vi "Send.vi"(9 "Nested Error":errorcluster, 10 "Nested Actor":refnum<class "Actor.lvclass">) -> (3 "Actor Last Ack Msg Strategy out":refnum<class "Actor Last Ack Msg Strategy.lvclass">)   [LabVIEW 2021, in "Actor Last Ack.lvlib" / "Actor Last Ack Msg Strategy.lvclass"]
uses:
  Actor Last Ack Msg Strategy.lvclass
  LVCAM/Actor/Actor.lvclass
  Actor Last Ack Msg Strategy.lvclass/Actor Last Ack Msg Strategy.ctl
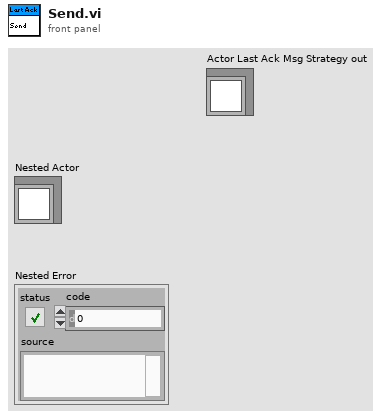
[diagram p1: front panel]
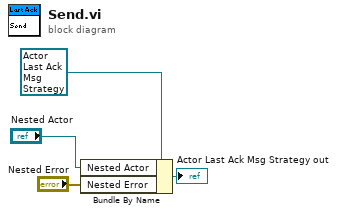
[diagram p0: block diagram]
diagram:
  n1 = Bundle By Name(cluster=refnum<class "Actor Last Ack Msg Strategy.lvclass"> refnum ("Last Ack Msg in"), "Nested Actor"="Nested Actor", "Nested Error"="Nested Error") -> (→"Actor Last Ack Msg Strategy out":refnum<class "Actor Last Ack Msg Strategy.lvclass">)
